vi "16.扫描引擎同步高阶.vi"() -> ()   [LabVIEW 2019]
uses:
  <vilib>/rvi/Emulation/niFpgaGetClockAttributes.vi
  <vilib>/rvi/Emulation/niFpgaSctlEmulationGetInTimedLoop.vi
  <vilib>/rvi/Emulation/niFpgaEmulationReportErrorSimple.vi
  <vilib>/rvi/eio/common/nirviEmuTemplatePropertyGet_noerrors.vi
  <vilib>/rvi/Emulation/niFpgaCriticalErrorInLSC.vi
  <vilib>/rvi/eio/common/nirviEmuTemplateMethod_errors.vi
  <vilib>/eio/EIOPropertyNode/EIOPropertyNode.xnode
  <vilib>/eio/EIOMethodNode/EIOMethodNode.xnode
  <vilib>/rvi/eio/common/nirviEmuTemplatePropertyGet_errors.vi
  <vilib>/rvi/eio/common/nirviEmuTemplatePropertySet_errors.vi
  <vilib>/rvi/eio/common/nirviEmuTemplatePropertySet_noerrors.vi
panel:
  in  "Stop":bool
  in  "Reset Missed Falling Edge Latch":bool
  out "Missed Falling Edge Latched":bool
  in  "Delay Time":u32
  out "Missed Falling Edge Instantaneous":bool
  out "Scan Clock High Time":u32
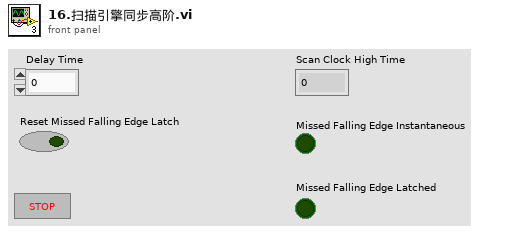
[diagram p1: front panel]
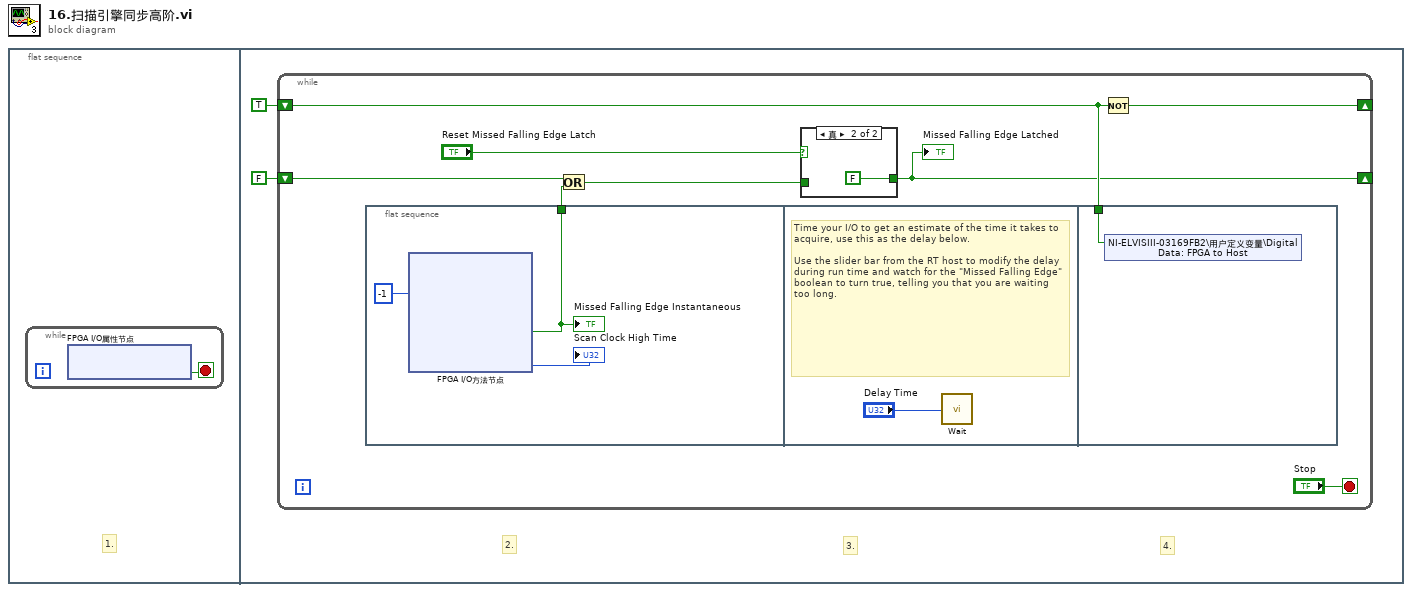
[diagram p0: block diagram]
diagram:
  n1 = flat-sequence {
    frame #0 {
      # "1."
      n2 = while {
        stop <- w1 stop-if-true
        n3 = xnode "FPGA I/O属性节点"() -> ("启用"=w1:bool)  [unwired: 1 in, 1 out]
      }
    }
    frame #1 {
      # "4."
      # "3."
      # "2."
      n4 = while {
        shift-right: [w11] -> _
        shift-left: TRUE -> [w10]
        shift-right: [w6] -> _
        shift-left: FALSE -> [w8]
        stop <- "Stop" stop-if-true
        n5 = flat-sequence {
          tunnel: [w13] -> w7
          tunnel: w10 -> [w16]
          frame #0 {
            n6 = xnode "FPGA I/O方法节点"("超时"=-1 ("Timeout")) -> ("丢失的下降沿"=w13:bool, "高时间"=→"Scan Clock High Time":u32)  [unwired: 1 in, 3 out]
            "Missed Falling Edge Instantaneous" <- w13
          }
          frame #1 {
            # "Time your I/O to get an estimate of the time it takes to acquire, use this as the delay below.\n\nUse the slider bar from the RT host to modify the delay during run time and watch for the \"Missed Falling Edge\" boolean to turn true, telling you that you are waiting too long."
            n7 = call "Wait"("Count(Ticks)"="Delay Time") -> ()  [unwired: 1 out]
          }
          frame #2 {
            n8 = shared-variable "NI-ELVISIII-03169FB2\\用户定义变量\\Digital Data: FPGA to Host"(w16) -> ()  [unwired: 1 in, 1 out]
          }
        }
        n9 = Or(x=w8, y=w7) -> (x .or. y?=w4:bool)
        n10 = case shown="真" "Reset Missed Falling Edge Latch" {
          tunnel: [w17 FALSE] -> w6
          tunnel: w4 -> [w17 _]
          frame False {
          }
          frame True {
          }
        }
        "Missed Falling Edge Latched" <- w6
        n11 = Not(x=w10) -> (.not. x?=w11:bool)
      }
    }
  }
